vi "Undo.vi"(8 "error in (no error)":errorcluster, 11 "UndoObject in":refnum<class "UndoObject.lvclass">) -> (0 "error out":errorcluster, 2 "Ctrl Val.Get All":T1[](array[typedef]), 3 "UndoObject out":refnum<class "UndoObject.lvclass">, 4 "Redo Enable":bool, 6 "Undo Enable":bool)   [LabVIEW 2015, in "UndoLibrary.lvlib" / "UndoObject.lvclass"]
doc: "This VI stores the values to perform the undo action."
uses:
  UndoObject.lvclass
  Support VIs/DataClass/Controls/cluster_Control Value.ctl
  UndoObject.lvclass/UndoObject.ctl
  Support VIs/DataClass/DataObject.lvclass/DataObject.ctl
  QueueOperations/QueueOperations.lvlib
  Support VIs/DataClass/DataObject.lvclass
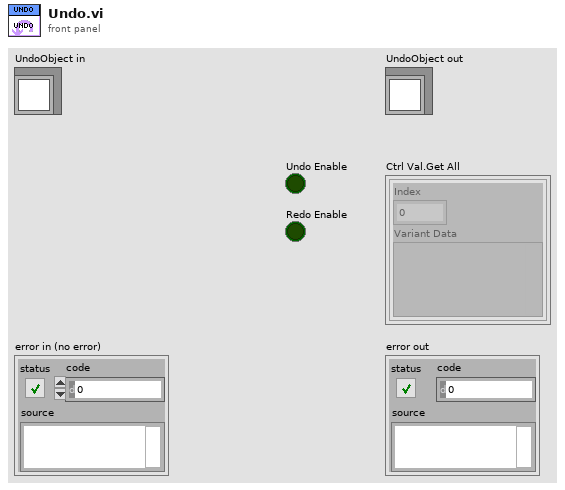
[diagram p1: front panel]
types:
  T1 = typedef "UndoLibrary.lvlib/DataObject.lvclass/cluster_Control Value.ctl" = cluster{"Index":i32, "Variant Data":variant}
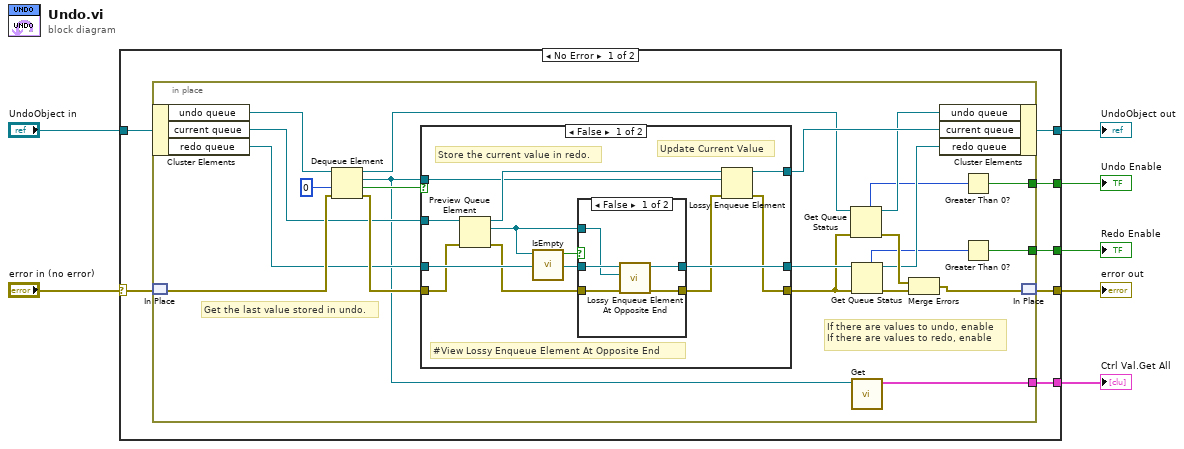
[diagram p0: block diagram]
diagram:
  n1 = case shown="No Error" "error in (no error)" {
    selector: "error in (no error)" -> [w14 w60]
    tunnel: [w13 w60] -> w7
    tunnel: "UndoObject in" -> [w12 w59]
    tunnel: [w11 w59] -> w2
    tunnel: [w10 _] -> w1
    tunnel: [w9 _] -> w5
    tunnel: [w8 _] -> w4
    frame No Error {
      n2 = in-place {
        in-place-border: [w15] -> w10
        in-place-border: [w19] -> w9
        in-place-border: [w17] -> w8
        # "Get the last value stored in undo."
        # "If there are values to undo, enable\nIf there are values to redo, enable"
        n3 = in-place-cluster #1(w12) -> ("undo queue"=w32:refnum<queue>, "current queue"=w31:refnum<queue>, "redo queue"=w30:refnum<queue>)
        n4 = in-place-match #2(w14) -> (w33:errorcluster)
        n5 = Dequeue Element(queue=w32, timeout in ms (-1)=0, error in (no error)=w33) -> (queue out=w23:refnum<queue>, element=w16:refnum<class "DataObject.lvclass">, timed out?=w36:bool, error out=w34:errorcluster)
        n6 = case shown="False" w36 {
          tunnel: w30 -> [w48 w58]
          tunnel: [w47 w58] -> w29
          tunnel: w16 -> [w41 _]
          tunnel: w31 -> [w46 w57]
          tunnel: w34 -> [w45 w56]
          tunnel: [w42 w57] -> w28
          tunnel: [w44 w56] -> w26
          frame False {
            # "Store the current value in redo."
            # "Update Current Value"
            # "#View Lossy Enqueue Element At Opposite End"
            n7 = Preview Queue Element(queue=w46, error in (no error)=w45) -> (queue out=w43:refnum<queue>, element=w38:refnum<class "DataObject.lvclass">, error out=w40:errorcluster)  [unwired: 1 in, 1 out]
            n8 = call "IsEmpty.vi"("DataObject in"=w38) -> ("empty?"=w37:bool)  [unwired: 9 in, 1 out]
            n9 = case shown="False" w37 {
              tunnel: w40 -> [w51 w54]
              tunnel: w48 -> [w53 w55]
              tunnel: [w50 w55] -> w47
              tunnel: [w49 w54] -> w39
              tunnel: w38 -> [w52 _]
              frame False {
                n10 = call "Lossy Enqueue Element At Opposite End.vi"("error in (no error)"=w51, "element"=w52, "queue in"=w53) -> ("error out"=w49:errorcluster, "queue out"=w50:refnum<queue>)  [unwired: 5 in, 2 out]
              }
              frame True {
              }
            }
            n11 = Lossy Enqueue Element(queue=w43, element=w41, error in (no error)=w39) -> (queue out=w42:refnum<queue>, error out=w44:errorcluster)  [unwired: 2 out]
          }
          frame True {
          }
        }
        n12 = Get Queue Status(queue=w23, error in (no error)=w26) -> (queue out=w22:refnum<queue>, error out=w24:errorcluster, # elements in queue=w20:i32)  [unwired: 1 in, 5 out]
        n13 = Get Queue Status(queue=w29, error in (no error)=w26) -> (queue out=w21:refnum<queue>, error out=w27:errorcluster, # elements in queue=w18:i32)  [unwired: 1 in, 5 out]
        n14 = call "Get.vi"("DataObject in"=w16) -> ("Conrol Value[]"=w15:T1[])  [unwired: 9 in, 1 out]
        n15 = Merge Errors(w24, w27) -> (w25:errorcluster)
        n16 = in-place-cluster #1("undo queue"=w22, "current queue"=w28, "redo queue"=w21) -> (w11:refnum<class "UndoObject.lvclass">)
        n17 = Greater Than 0?(x=w20) -> (x > 0?=w19:bool)
        n18 = Greater Than 0?(x=w18) -> (x > 0?=w17:bool)
        n19 = in-place-match #2(w25) -> (w13:errorcluster)
      }
    }
    frame Error {
    }
  }
  "error out" <- w7
  "Ctrl Val.Get All" <- w1
  "Undo Enable" <- w5
  "Redo Enable" <- w4
  "UndoObject out" <- w2
